vi "Continuous Random.vi"   [LabVIEW 2017, in "NI_Gmath.lvlib"]
doc: "Generates random values from a variate X, where X describes the selected distribution type. You must manually select the polymorphic instance to use."
uses:
  <vilib>/gmath/NI_Gmath.lvlib
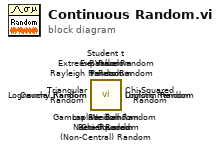
[diagram p0: block diagram]
diagram:
  n1 = call <vilib>:"Laplace Random.vi"() -> ()  [unwired: 10 in, 2 out]
  n2 = call <vilib>:"Pareto Random.vi"() -> ()  [unwired: 10 in, 2 out]
  n3 = call <vilib>:"Lognormal Random.vi"() -> ()  [unwired: 10 in, 2 out]
  n4 = call <vilib>:"Logistic Random.vi"() -> ()  [unwired: 10 in, 2 out]
  n5 = call <vilib>:"Chi-Squared (Non-Central) Random.vi"() -> ()  [unwired: 10 in, 2 out]
  n6 = call <vilib>:"Extreme Value Random.vi"() -> ()  [unwired: 10 in, 2 out]
  n7 = call <vilib>:"Rayleigh Random.vi"() -> ()  [unwired: 10 in, 2 out]
  n8 = call <vilib>:"Weibull Random.vi"() -> ()  [unwired: 10 in, 2 out]
  n9 = call <vilib>:"Uniform Random.vi"() -> ()  [unwired: 10 in, 2 out]
  n10 = call <vilib>:"Triangular Random.vi"() -> ()  [unwired: 10 in, 2 out]
  n11 = call <vilib>:"Student t Random.vi"() -> ()  [unwired: 10 in, 2 out]
  n12 = call <vilib>:"Normal Random.vi"() -> ()  [unwired: 10 in, 2 out]
  n13 = call <vilib>:"Gamma Random.vi"() -> ()  [unwired: 10 in, 2 out]
  n14 = call <vilib>:"F Random.vi"() -> ()  [unwired: 10 in, 2 out]
  n15 = call <vilib>:"Exp Random.vi"() -> ()  [unwired: 10 in, 2 out]
  n16 = call <vilib>:"Chi-Squared Random.vi"() -> ()  [unwired: 10 in, 2 out]
  n17 = call <vilib>:"Cauchy Random.vi"() -> ()  [unwired: 10 in, 2 out]
  n18 = call <vilib>:"Beta Random.vi"() -> ()  [unwired: 10 in, 2 out]
